vi "bloc_turbodecodage.vi"(10 "sigma2":string, 11 "Array":cdb[](array[numeric])) -> (1 "sortie complexe":string, 2 "sortie décodeur":string, 3 "output bit stream":i8[](array[numeric]))   [LabVIEW 2018]
uses:
  <vilib>/addons/Modulation/niDMT.lvlib
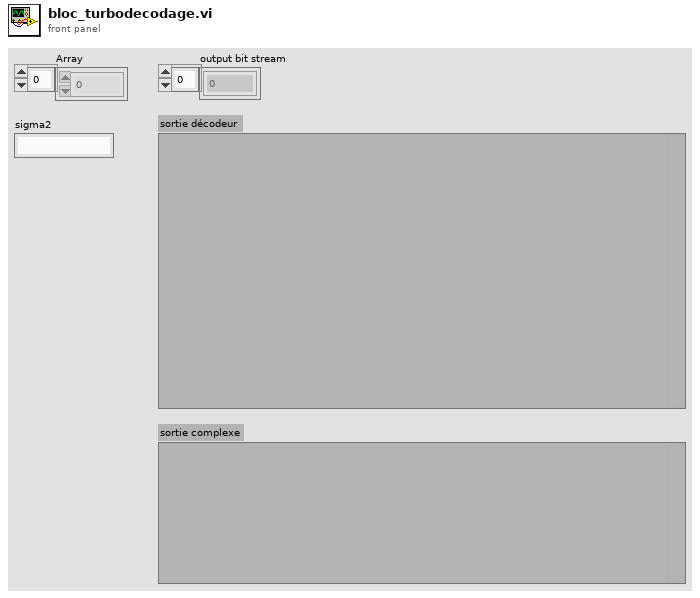
[diagram p1: front panel]
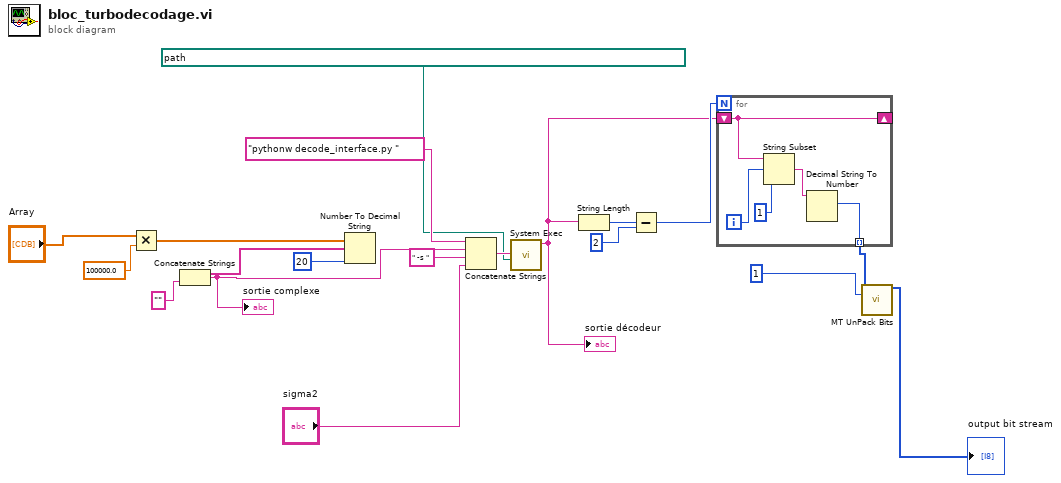
[diagram p0: block diagram]
diagram:
  n1 = Multiply(x="Array", y=100000.0 ("x")) -> (x*y=w15:cdb[])
  n2 = Number To Decimal String(number=w15, width (-)=i16 20) -> (decimal integer string=w19:string[])
  n3 = Concatenate Strings(w19, "") -> (w13:string)
  "sortie complexe" <- w13
  n4 = Concatenate Strings("pythonw decode_interface.py ", w13, " -s " ("string"), "sigma2") -> (w12:string)
  n5 = call <vilib>:"System Exec.vi"("working directory"=path "C:/Users/pc-labview/Desktop/Levi/Turbo-Codes/Implémentation perso Python/Turbocodes_OO", "command line"=w12) -> ("standard output"=w3:string)  [unwired: 4 in, 5 out]
  "sortie décodeur" <- w3
  n6 = String Length(string=w3) -> (length=w6:i32)
  n7 = Subtract(x=w6, y=2) -> (x-y=w4:i32)
  n8 = for {
    N: w4 -> [_]
    tunnel: [w21] -> w7 mode=indexing
    shift-right: [w20] -> _
    shift-left: w3 -> [w20]
    i -> [w24]
    n9 = String Subset(string=w20, offset (0)=w24, length (rest)=1) -> (substring=w22:string)
    n10 = Decimal String To Number(string=w22) -> (number=w21:i32)  [unwired: 2 in, 1 out]
  }
  n11 = call <vilib>:"MT UnPack Bits.vi"("input integers"=w7, "bits per integer"=1) -> ("output bit stream"=→"output bit stream":i8[])  [unwired: 12 in, 1 out]
